vi "tab init.vi"() -> (0 "Image 3":T1(plugin-control), 1 "Image 2":T1(plugin-control), 2 "Image":T1(plugin-control), 3 "appended array":string[][](array[string]), 4 "Image 4":T1(plugin-control))   [LabVIEW 2019]
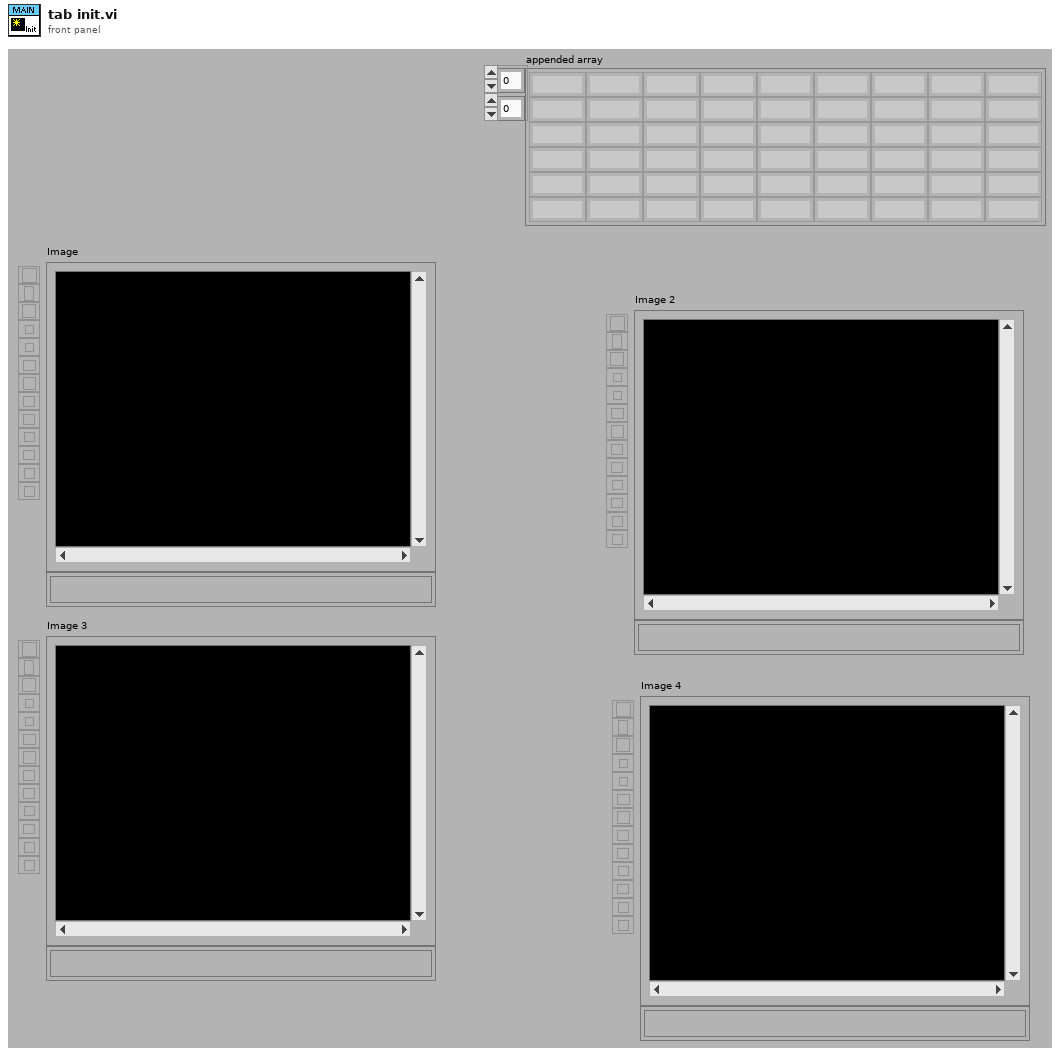
[diagram p1: front panel]
types:
  T1 = typedef "IMAQ Image.ctl" = refnum<image>
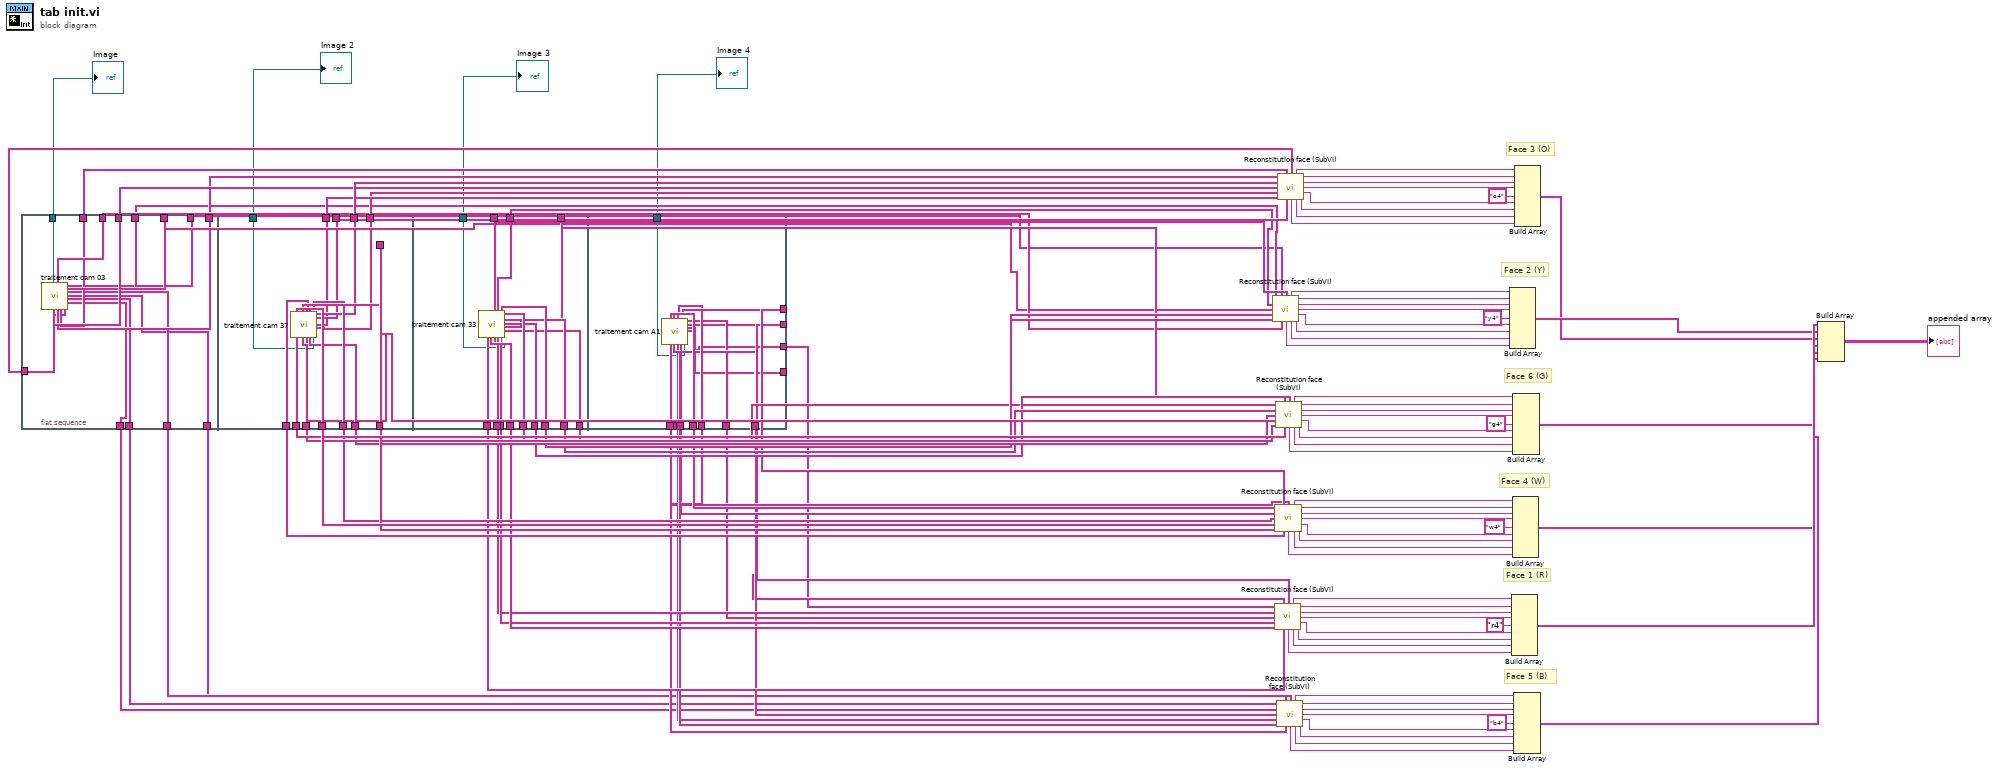
[diagram p0: block diagram]
diagram:
  # "Face 6 (G)"
  # "Face 5 (B)"
  # "Face 4 (W)"
  # "Face 3 (O)"
  # "Face 2 (Y)"
  # "Face 1 (R)"
  n1 = flat-sequence {
    tunnel: [w126] -> w16
    tunnel: [w125] -> w15
    tunnel: [w124] -> w14
    tunnel: [w123] -> w13
    tunnel: [w122] -> w12
    tunnel: [w121] -> w11
    tunnel: [w120] -> w10
    tunnel: [w119] -> w9
    tunnel: [w118] -> w8
    tunnel: [w117] -> w7
    tunnel: [w116] -> w6
    tunnel: [w115] -> w5
    tunnel: [w114] -> w4
    tunnel: [w139] -> w52
    tunnel: [w138] -> w51
    tunnel: [w137] -> w50
    tunnel: [w136] -> w49
    tunnel: [w135] -> w48
    tunnel: [w128] -> w47
    tunnel: [w134] -> w46
    tunnel: [w133] -> w45
    tunnel: [w132] -> w44
    tunnel: [w131] -> w43
    tunnel: [w130] -> w42
    tunnel: [w129] -> w41
    tunnel: [w127] -> w3
    tunnel: [w152] -> w40
    tunnel: [w151] -> w39
    tunnel: [w150] -> w38
    tunnel: [w149] -> w37
    tunnel: [w148] -> w36
    tunnel: [w147] -> w35
    tunnel: [w146] -> w34
    tunnel: [w145] -> w33
    tunnel: [w144] -> w32
    tunnel: [w143] -> w31
    tunnel: [w142] -> w30
    tunnel: [w141] -> w29
    tunnel: [w140] -> w2
    tunnel: [w165] -> w28
    tunnel: [w164] -> w27
    tunnel: [w163] -> w26
    tunnel: [w162] -> w25
    tunnel: [w161] -> w24
    tunnel: [w160] -> w23
    tunnel: [w159] -> w22
    tunnel: [w158] -> w21
    tunnel: [w157] -> w20
    tunnel: [w156] -> w19
    tunnel: [w155] -> w18
    tunnel: [w154] -> w17
    tunnel: [w153] -> w1
    frame #0 {
      n2 = call "traitement cam 03.vi"() -> ("Image Out"=w114:T1, "Couleur carré 12 (3,6)"=w126:string[], "Couleur carré 4 (2,9)"=w125:string[], "Couleur carré 9 (3,3)"=w124:string[], "Couleur carré 3 (2,6)"=w123:string[], "Couleur carré 10 (3,2)"=w122:string[], "Couleur carré 2 (2,3)"=w121:string[], "Couleur carré 11 (3,1)"=w115:string[], "Couleur carré 1 (2,2)"=w120:string[], "Couleur carré 6 (5,1)"=w119:string[], "Couleur carré 7 (5,2)"=w118:string[], "Couleur carré 8 (5,3)"=w117:string[], "Couleur carré 5 (5,4)"=w116:string[])  [unwired: 14 in, 1 out]
    }
    frame #1 {
      n3 = call "traitement cam 37.vi"() -> ("Couleur carré 8 (4,7)"=w139:string[], "Couleur carré 11 (6,9)"=w138:string[], "Couleur carré 7 (4,8)"=w137:string[], "Couleur carré 10 (6,8)"=w136:string[], "Couleur carré 6 (4,9)"=w135:string[], "Couleur carré 9 (6,7)"=w128:string[], "Couleur carré 5 (4,6)"=w134:string[], "Couleur carré 12 (6,6)"=w133:string[], "Image Out"=w127:T1, "Couleur carré 1 (3,4)"=w132:string[], "Couleur carré 2 (3,9)"=w131:string[], "Couleur carré 3 (3,8)"=w130:string[], "Couleur carré 4 (3,7)"=w129:string[])  [unwired: 14 in, 1 out]
    }
    frame #2 {
      n4 = call "traitement cam 33.vi"() -> ("Couleur carré 11 (1,9)"=w152:string[], "Couleur carré 10  (1,8)"=w151:string[], "Couleur carré 4 (2,1)"=w150:string[], "Couleur carré 9 (1,7)"=w149:string[], "Couleur carré 3 (2,4)"=w148:string[], "Couleur carré 12 (1,4)"=w147:string[], "Couleur carré 2 (2,7)"=w146:string[], "Image Out"=w140:T1, "Couleur carré 1 (2,8)"=w145:string[], "Couleur carré 5 (6,4)"=w144:string[], "Couleur carré 6 (6,1)"=w143:string[], "Couleur carré 7 (6,2)"=w142:string[], "Couleur carré 8 (6,3)"=w141:string[])  [unwired: 14 in, 1 out]
    }
    frame #3 {
      n5 = call "traitement cam A1.vi"() -> ("Couleur carré 8 (4,3)"=w165:string[], "Couleur carré 11 (5,9)"=w164:string[], "Couleur carré 7 (4,2)"=w163:string[], "Couleur carré 10 (5,8)"=w162:string[], "Couleur carré 6 (4,1)"=w161:string[], "Couleur carré 9 (5,7)"=w160:string[], "Couleur carré 5 (4,4)"=w159:string[], "Couleur carré 12 (5,6)"=w158:string[], "Image Out"=w153:T1, "Couleur carré 1 (1,6)"=w157:string[], "Couleur carré 2 (1,1)"=w156:string[], "Couleur carré 3 (1,2)"=w155:string[], "Couleur carré 4 (1,3)"=w154:string[])  [unwired: 14 in, 1 out]
    }
  }
  n6 = call "Reconstitution face (SubVI).vi"("Couleur carrée  2"=w11, "Couleur carrée  1"=w10, "Couleur carrée 0"=w38, "Couleur carrée  3"=w36, "Couleur carrée  5"=w13, "Couleur carrée  6"=w34, "Couleur carrée  7"=w33, "Couleur carrée  8"=w15) -> ("Couleur 0"=w96:string, "Couleur 1"=w97:string, "Couleur  2"=w98:string, "Couleur 3"=w99:string, "Couleur 5"=w100:string, "Couleur 8"=w102:string, "Couleur 7"=w103:string, "Couleur 6"=w101:string)
  n7 = call "Reconstitution face (SubVI).vi"("Couleur carrée  2"=w17, "Couleur carrée  1"=w18, "Couleur carrée 0"=w19, "Couleur carrée  3"=w35, "Couleur carrée  5"=w20, "Couleur carrée  6"=w37, "Couleur carrée  7"=w39, "Couleur carrée  8"=w40) -> ("Couleur 0"=w113:string, "Couleur 1"=w112:string, "Couleur  2"=w111:string, "Couleur 3"=w110:string, "Couleur 5"=w109:string, "Couleur 8"=w107:string, "Couleur 7"=w106:string, "Couleur 6"=w108:string)
  n8 = call "Reconstitution face (SubVI).vi"("Couleur carrée  2"=w28, "Couleur carrée  1"=w26, "Couleur carrée 0"=w24, "Couleur carrée  3"=w22, "Couleur carrée  5"=w46, "Couleur carrée  6"=w52, "Couleur carrée  7"=w50, "Couleur carrée  8"=w48) -> ("Couleur 0"=w78:string, "Couleur 1"=w79:string, "Couleur  2"=w80:string, "Couleur 3"=w81:string, "Couleur 5"=w82:string, "Couleur 8"=w84:string, "Couleur 7"=w85:string, "Couleur 6"=w83:string)
  n9 = call "Reconstitution face (SubVI).vi"("Couleur carrée  2"=w29, "Couleur carrée  1"=w30, "Couleur carrée 0"=w31, "Couleur carrée  3"=w32, "Couleur carrée  5"=w45, "Couleur carrée  6"=w47, "Couleur carrée  7"=w49, "Couleur carrée  8"=w51) -> ("Couleur 0"=w60:string, "Couleur 1"=w61:string, "Couleur  2"=w62:string, "Couleur 3"=w63:string, "Couleur 5"=w64:string, "Couleur 8"=w66:string, "Couleur 7"=w67:string, "Couleur 6"=w65:string)
  n10 = call "Reconstitution face (SubVI).vi"("Couleur carrée  2"=w7, "Couleur carrée  1"=w8, "Couleur carrée 0"=w9, "Couleur carrée  3"=w6, "Couleur carrée  5"=w21, "Couleur carrée  6"=w23, "Couleur carrée  7"=w25, "Couleur carrée  8"=w27) -> ("Couleur 0"=w77:string, "Couleur 1"=w76:string, "Couleur  2"=w75:string, "Couleur 3"=w74:string, "Couleur 5"=w73:string, "Couleur 8"=w71:string, "Couleur 7"=w70:string, "Couleur 6"=w72:string)
  n11 = call "Reconstitution face (SubVI).vi"("Couleur carrée  2"=w14, "Couleur carrée  1"=w12, "Couleur carrée 0"=w5, "Couleur carrée  3"=w44, "Couleur carrée  5"=w16, "Couleur carrée  6"=w41, "Couleur carrée  7"=w42, "Couleur carrée  8"=w43) -> ("Couleur 0"=w95:string, "Couleur 1"=w94:string, "Couleur  2"=w93:string, "Couleur 3"=w92:string, "Couleur 5"=w91:string, "Couleur 8"=w89:string, "Couleur 7"=w88:string, "Couleur 6"=w90:string)
  n12 = Build Array(w96, w97, w98, w99, "y4" ("element"), w100, w101, w103, w102) -> (w58:string[])
  n13 = Build Array(w113, w112, w111, w110, "r4" ("element"), w109, w108, w106, w107) -> (w59:string[])
  n14 = Build Array(w78, w79, w80, w81, "w4" ("element"), w82, w83, w85, w84) -> (w56:string[])
  n15 = Build Array(w60, w61, w62, w63, "g4" ("element"), w64, w65, w67, w66) -> (w54:string[])
  n16 = Build Array(w77, w76, w75, w74, "b4" ("element"), w73, w72, w70, w71) -> (w55:string[])
  n17 = Build Array(w95, w94, w93, w92, "o4" ("element"), w91, w90, w88, w89) -> (w57:string[])
  n18 = Build Array(w59, w58, w57, w56, w55, w54) -> (→"appended array":string[][])
  "Image" <- w4
  "Image 2" <- w3
  "Image 3" <- w2
  "Image 4" <- w1
